vi "global_variables.vi"() -> ()   [LabVIEW 2015]
uses:
  Classes/AnalysisList/AnalysisList.lvclass
  MSControl/Classes/Plots/Plots.lvclass
panel:
  in  "PlotObjectsQueue":refnum<queue>
  in  "DataSource":string
  in  "export folder":path
  in  "source folder":path
  in  "AnalysisList.lvclass":refnum<class "AnalysisList.lvclass">
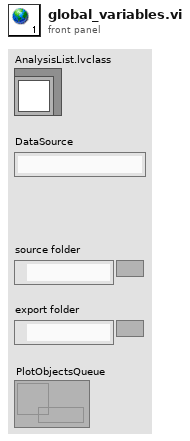
[diagram p1: front panel]
diagram:
